vi "CurrentController.vi"(0 "I_setpt":sgl format="%#_13g", 5 "I_procVar":sgl[](array[numeric])=[0.0, 0.0, 0.0, 0.0], 13 "settings":T1={"numberOfInterleaves"="", "rampRate"="", "manualInput"="", "perturbAmp"="", "perturbAngleInc"="", "reset"="", "state"="", "gains"="", "Currents"="Currents"}) -> (4 "output":sgl[](array[numeric]), 15 "perturbance":sgl)   [LabVIEW 2017, in "BuckBoost.lvlib"]
uses:
  BuckBoost.lvlib
  contSettings.ctl
  <vilib>/rvi/Analysis/control/PID/Typedef/niFpgaPID_PIState.ctl
  contState.ctl
  <vilib>/rvi/Analysis/control/PID/Typedef/niFpgaPID_ManualControl.ctl
  <vilib>/rvi/Analysis/control/PID/Typedef/niFpgaPID_OutputRange.ctl
  <vilib>/rvi/FXPMathLib/FxpSinAndCos/subVIs/nifxpmath_SinAndCos_SimConfig.ctl
  <vilib>/Utility/error.llb/Clear Errors.vi
  <vilib>/rvi/Emulation/niFpgaSctlEmulationGetInTimedLoop.vi
  <vilib>/rvi/DataTransferAndStorage/Container/Common/niFpgaContainerExecOnDevCompGetState.vi
  <vilib>/rvi/Emulation/niFpgaEmulationIsFPGAContextNoSignature.vi
  <vilib>/rvi/DataTransferAndStorage/Container/Common/niFpgaContainerGetUniqueNameForEmu.vi
  <vilib>/rvi/Memory/Memory_Emulation/niFpgaMemoryEmulationCacheClearOnFirstRun.vi
  <vilib>/rvi/Memory/Memory_Emulation/nirvimemoryEmulationManagerCache_MakeExclusive.vi
  <vilib>/rvi/Memory/Memory_Emulation/niFpgaMemoryEmulationValidateCache.vi
  <vilib>/rvi/Memory/Memory_Emulation/nirvimemoryEmulationManagerCache_InsertValue.vi
  <vilib>/rvi/Memory/Memory_Emulation/nirvimemoryEmulationManagerCache_ReleaseExclusive.vi
  <vilib>/rvi/Memory/Memory_Emulation/nirvimemoryEmulationManagerCache_GetValue.vi
  <vilib>/rvi/Memory/Memory_Emulation/nirvimemoryEmulationManagerCache_SetValue.vi
  <vilib>/rvi/Emulation/niFpgaProcessEmulError.vi
  <vilib>/rvi/FXPMathLib/FxpSinAndCos/simVIs/DllFxpSinAndCosTemp_sub.vi
  <userlib>/_NI FLP Library/FPGA/outsideSCTL/FlpLib Multiply Shared Instance 0.vi
  <userlib>/_NI FLP Library/addons/Control/Ramp/FlpLib Ramp 0.vi
  <userlib>/_NI FLP Library/FPGA/outsideSCTL/FlpLib Subtract Shared Instance 0.vi
  <userlib>/_NI FLP Library/addons/Control/PI_Controller/FlpLib PI_Controller 0.vi
  <vilib>/rvi/DataTransferAndStorage/Container/XNode/niFpgaContainer.xnode
  <vilib>/rvi/DataTransferAndStorage/Register/Emulation/niFpgaRegisterEmulationRefIn.vi
  <vilib>/rvi/FXPMathLib/FxpSinAndCos/XNode/nifxpmath_SinAndCos.xnode
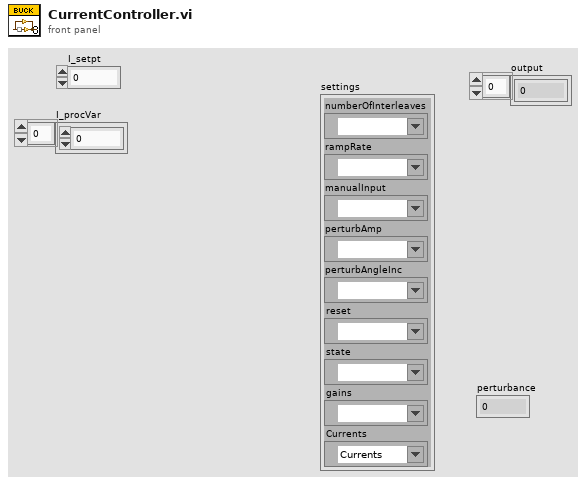
[diagram p1: front panel]
types:
  T1 = typedef "BuckBoost.lvlib/contSettings.ctl" = cluster{"numberOfInterleaves":refnum<k21>, "rampRate":refnum<k21>, "manualInput":refnum<k21>, "perturbAmp":refnum<k21>, "perturbAngleInc":refnum<k21>, "reset":refnum<k21>, "state":refnum<k21>, "gains":refnum<k21>, "Currents":refnum<k21>}
  T2 = typedef "niFpgaPID_OutputRange.ctl" = cluster{"output high (Inf)":sgl, "output low (-Inf)":sgl}
  T3 = typedef "BuckBoost.lvlib/contState.ctl" = enum16{"disabled", "manual", "normal", "perturb"}
  T4 = typedef "niFpgaPID_ManualControl.ctl" = cluster{"manual? (F)":bool, "manual input (0)":sgl}
  T5 = typedef "niFpgaPID_PIState.ctl" = cluster{"uI(k-1)":sgl, "e(k-1)":sgl, "output (k-1)":sgl}
  T6 = enum16{"disabled", "manual", "normal", "perturb"}
  T7 = cluster{"proportional gain":sgl, "integral gain":sgl}
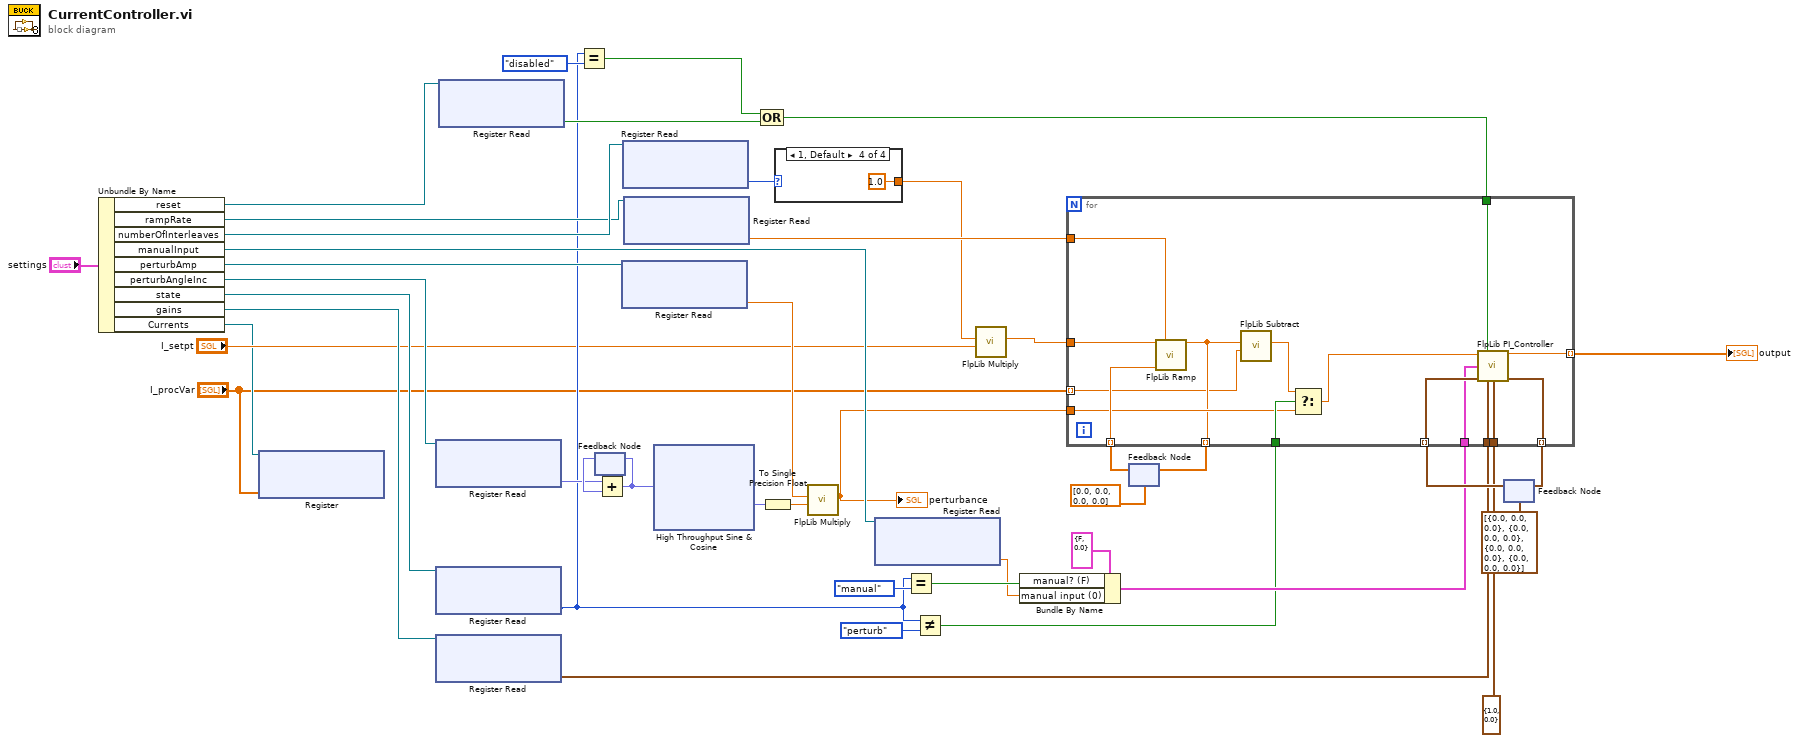
[diagram p0: block diagram]
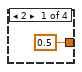
[diagram p2: hidden frame]
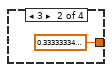
[diagram p3: hidden frame]
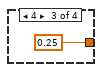
[diagram p4: hidden frame]
diagram:
  n1 = Unbundle By Name("settings") -> ("reset"=w15:refnum<k21>, "rampRate"=w22:refnum<k21>, "numberOfInterleaves"=w24:refnum<k21>, "manualInput"=w20:refnum<k21>, "perturbAmp"=w18:refnum<k21>, "perturbAngleInc"=w17:refnum<k21>, "state"=w13:refnum<k21>, "gains"=w11:refnum<k21>, "Currents"=w2:refnum<k21>)
  n2 = xnode "Register"("Data"="I_procVar", "Register In"=w2) -> ()  [unwired: 1 out]
  n3 = xnode ("Register Read")("Register In"=w17) -> ("Data"=w16:fxp<+/-,16,0>)  [unwired: 1 out]
  n4 = xnode ("Register Read")("Register In"=w13) -> ("Data"=w12:T6)  [unwired: 1 out]
  n5 = xnode ("Register Read")("Register In"=w11) -> ("Data"=w10:T7)  [unwired: 1 out]
  n6 = xnode ("Register Read")("Register In"=w15) -> ("Data"=w14:bool)  [unwired: 1 out]
  n7 = Equal?(x=w12, y=contState."disabled") -> (x = y?=w26:bool)
  n8 = feedback #1() -> (w33:fxp<+/-,16,1>)  [unwired: 1 in]
  n9 = Add(x=w16, y=w33) -> (x+y=w32:fxp<+/-,16,1>)
  n10 = feedback-in #1(w32) -> ()
  n11 = xnode ("Register Read")("Register In"=w18) -> ("Data"=w9:sgl)  [unwired: 1 out]
  n12 = xnode ("Register Read")("Register In"=w24) -> ("Data"=w23:u8)  [unwired: 1 out]
  n13 = xnode ("Register Read")("Register In"=w22) -> ("Data"=w21:sgl)  [unwired: 1 out]
  n14 = xnode "High Throughput Sine & Cosine"("x (pi)"=w32) -> ("sin(x)"=w3:fxp<+/-,16,2>)  [unwired: 1 out]
  n15 = Compound Arithmetic op=OR(w26, w14) -> (w25:bool)
  n16 = To Single Precision Float(number=w3) -> (single precision float=w4:sgl)
  n17 = case shown="1, Default" w23 {
    tunnel: [sgl 0.5 sgl 0.33333334 sgl 0.25 sgl 1.0] -> w6
    frame 2 {
    }
    frame 3 {
    }
    frame 4 {
    }
    frame 1, Default {
    }
  }
  n18 = call-poly <userlib>:"FlpLib Multiply.vi"("y"=w4, "x"=w9) -> ("x*y"=w8:sgl)  [unwired: 5 in]
  "perturbance" <- w8
  n19 = xnode ("Register Read")("Register In"=w20) -> ("Data"=w19:sgl)  [unwired: 1 out]
  n20 = Equal?(x=w12, y=contState."manual") -> (x = y?=w29:bool)
  n21 = Not Equal?(x=w12, y=contState."perturb") -> (x != y?=w28:bool)
  n22 = call-poly <userlib>:"FlpLib Multiply.vi"("y"="I_setpt", "x"=w6) -> ("x*y"=w7:sgl)  [unwired: 5 in]
  n23 = Bundle By Name(cluster=T4 {"manual? (F)"=FALSE, "manual input (0)"=0.0} ("manual control"), "manual? (F)"=w29, "manual input (0)"=w19) -> (w34:T4)
  n24 = feedback #2(sgl[] [0.0, 0.0, 0.0, 0.0]) -> (w37:sgl[])
  n25 = feedback #3(T5[] [{"uI(k-1)"=0.0, "e(k-1)"=0.0, "output (k-1)"=0.0}, {"uI(k-1)"=0.0, "e(k-1)"=0.0, "output (k-1)"=0.0}, {"uI(k-1)"=0.0, "e(k-1)"=0.0, "output (k-1)"=0.0}, {"uI(k-1)"=0.0, "e(k-1)"=0.0, "output (k-1)"=0.0}]) -> (w42:T5[])
  n26 = for {
    tunnel: [w64] -> w44 mode=indexing
    tunnel: w42 -> [w63] mode=indexing
    tunnel: w25 -> [w62]
    tunnel: [w53] -> w41 mode=indexing
    tunnel: w7 -> [w61]
    tunnel: "I_procVar" -> [w50] mode=indexing
    tunnel: [w52] -> w39 mode=indexing
    tunnel: w37 -> [w60] mode=indexing
    tunnel: w21 -> [w59]
    tunnel: w10 -> [w58]
    tunnel: T2 {"output high (Inf)"=1.0, "output low (-Inf)"=0.0} ("output range") -> [w57]
    tunnel: w34 -> [w56]
    tunnel: w8 -> [w54]
    tunnel: w28 -> [w55]
    n27 = call-poly <userlib>:"FlpLib Ramp.vi"("input"=w61, "rampRate"=w59, "stateIn"=w60) -> ("output"=w52:sgl)  [unwired: 12 in]
    n28 = call-poly <userlib>:"FlpLib Subtract.vi"("y"=w50, "x"=w52) -> ("x-y"=w51:sgl)  [unwired: 5 in]
    n29 = Select(t=w51, s=w55, f=w54) -> (s? t:f=w49:sgl)
    n30 = call-poly <userlib>:"FlpLib PI_Controller.vi"("error"=w49, "reset? (F)"=w62, "manual control"=w56, "state in"=w63, "gains"=w58, "output range"=w57) -> ("output"=w53:sgl, "state out"=w64:T5)  [unwired: 6 in, 2 out]
  }
  "output" <- w41
  n31 = feedback-in #2(w39) -> ()
  n32 = feedback-in #3(w44) -> ()
